vi "Application Processes Path.vi"() -> (3 "Application Processes Path":path)   [LabVIEW 2019]
uses:
  <vilib>/Utility/sysdir.llb/System Directory Type.ctl
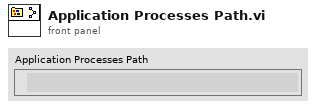
[diagram p1: front panel]
types:
  T1 = typedef "System Directory Type.ctl" = i32
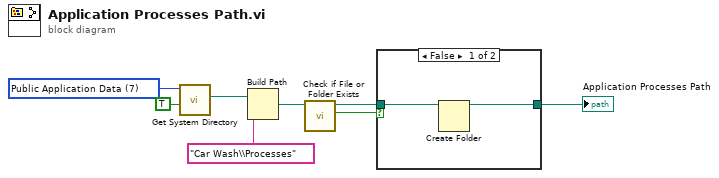
[diagram p0: block diagram]
diagram:
  w8 = T1 7 items=["User Home"=0, "User Desktop"=1, "User Documents"=2, "User Application Data"=3, "User Preferences"=4, "User Temporary"=5, "Public Documents"=6, "Public Application Data"=7, "Public Preferences"=8, "Public Cache"=13, "System Core Libraries"=9, "System Installed Libraries"=10, "Application Files"=11, "Boot Volume Root"=12] ("system directory type")
  n1 = call <vilib>:"Get System Directory.vi"("create directory if not found? (F)"=TRUE, "system directory type"=w8) -> ("system directory"=w6:path)  [unwired: 9 in]
  n2 = Build Path(base path=w6, name or relative path="Car Wash\\Processes") -> (appended path=w4:path)
  n3 = call <vilib>:"Check if File or Folder Exists.vi"("path"=w4) -> ("file or folder exists?"=w3:bool, "dup path"=w2:path)  [unwired: 8 in, 1 out]
  n4 = case shown="False" w3 {
    tunnel: w2 -> [w10 w11]
    tunnel: [w9 w11] -> w1
    frame False {
      n5 = Create Folder(path (use dialog)=w10) -> (created path=w9:path)  [unwired: 2 in, 2 out]
    }
    frame True {
    }
  }
  "Application Processes Path" <- w1
